vi "多刻度图表.vi"() -> ()   [LabVIEW 2010]
uses:
  <vilib>/Analysis/NI_AALBase.lvlib
panel:
  out "波形图表":dbl[][](graph)
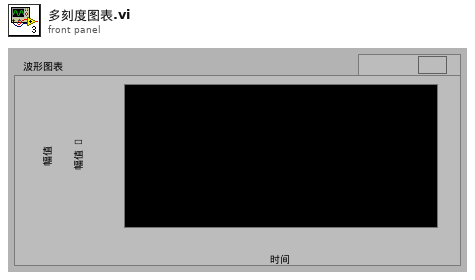
[diagram p1: front panel]
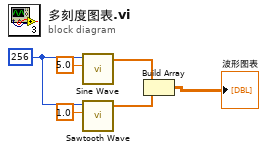
[diagram p0: block diagram]
diagram:
  w4 = 256
  n1 = call <vilib>:"Sine Wave.vi"("samples"=w4, "amplitude"=5.0) -> ("sine wave"=w6:dbl[])  [unwired: 3 in, 2 out]
  n2 = call <vilib>:"Sawtooth Wave.vi"("samples"=w4, "amplitude"=1.0) -> ("sawtooth wave"=w5:dbl[])  [unwired: 3 in, 2 out]
  n3 = Build Array(w6, w5) -> (→"波形图表":dbl[][])
